vi "DelayTest.vi"() -> ()   [LabVIEW 2018]
uses:
  Control/SSL UDP Address.ctl
panel:
  out "x":sgl
  in  "UDP RX":T1={"Port:"=10020, "Server IP:"="224.5.23.2", "Local IP:"="224.5.23.2", "RX"=FALSE}
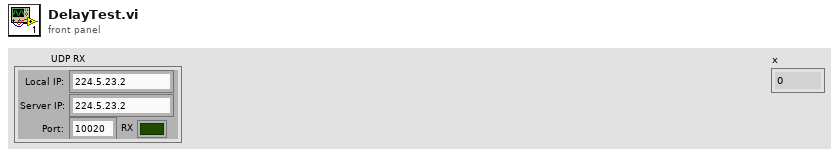
[diagram p1: front panel]
types:
  T1 = typedef "SSL UDP Address.ctl" = cluster{"Port:":u16, "Server IP:":string, "Local IP:":string, "RX":bool}
  T2 = typedef "VSS Detection Frame.ctl" = cluster{"robots_yellow":T3[], "robots_blue":T3[], "balls":T5[], "Valid":bool, "Time Stamp":timestamp}
  T3 = typedef "SSL Detection Robot.ctl" = cluster{"x":sgl, "robot_id":u32, "confidence":sgl, "y":sgl, "orientation":sgl, "pixel_x":sgl, "pixel_y":sgl, "height":sgl, "Valid":bool, "Time Stamp":timestamp, "x_k|k":T4, "Pk|k":T4, "Previous Time Stamp":timestamp, "R":T4}
  T4 = typedef "NI_Matrix.lvlib/RealMatrix.ctl" = dbl[][]
  T5 = typedef "SSL Detection Ball.ctl" = cluster{"x":sgl, "area":u32, "confidence":sgl, "y":sgl, "z":sgl, "pixel_x":sgl, "pixel_y":sgl, "Valid":bool, "Time Stamp":timestamp, "x_k|k":T4, "Pk|k":T4, "Id":u32, "Previous Time Stamp":timestamp, "R":T4}
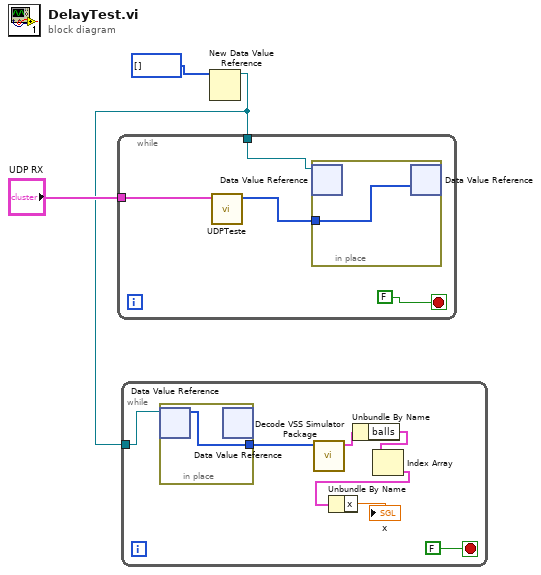
[diagram p0: block diagram]
diagram:
  n1 = New Data Value Reference(data value=u8[] [] ("data camera 2")) -> (data value reference=w1:refnum<data-value>)  [unwired: 1 in, 1 out]
  n2 = while {
    tunnel: "UDP RX" -> [w7]
    tunnel: w1 -> [w4]
    stop <- FALSE stop-if-true
    n3 = call "UDPTeste.vi"("UDP RX"=w7) -> ("data camera"=w5:u8[])  [unwired: 9 in, 1 out]
    n4 = in-place {
      in-place-border: w5 -> [w8]
      n5 = in-place-dvr #1(w4) -> ()  [unwired: 2 out]
      n6 = in-place-dvr #1(w8) -> ()  [unwired: 2 out]
    }
  }
  n7 = while {
    tunnel: w1 -> [w15]
    stop <- FALSE stop-if-true
    n8 = in-place {
      in-place-border: [w16] -> w13
      n9 = in-place-dvr #2(w15) -> (w16:u8[])  [unwired: 1 out]
      n10 = in-place-dvr #2() -> ()  [unwired: 1 in, 2 out]
    }
    n11 = call "Decode VSS Simulator Package.vi"("unsigned byte array"=w13) -> ("Detection Frame"=w12:T2)  [unwired: 9 in, 1 out]
    n12 = Unbundle By Name(w12) -> ("balls"=w11:T5[])
    n13 = Index Array(array=w11) -> (element=w10:T5)  [unwired: 1 in]
    n14 = Unbundle By Name(w10) -> ("x"=→"x":sgl)
  }
